vi "GUI_Ch300.vi"() -> ()   [LabVIEW 2013]
uses:
  Shared/GUI_Template/GUI_master/tcp_new_data_event.ctl
  Shared/GUI_Template/GUI_master/tcp new data cluster.ctl
  <vilib>/vision/NI_Vision_Development_Module.lvlib
panel:
  out "tcp data event":T1
  in  "Refresh Button":bool
  in  "localsavingpath::1":path caption="LocalSavingPath"
  in  "STOP":bool
  out "Lineout":dbl[](graph)
  in  "exposure::1":dbl=40.0 caption="Exposure" min=0.0 max=200.0
  in  "ADCGain::1":dbl=1.0 caption="ADC Gain" min=0.0 max=2000.0
  in  "save::1":bool caption="Save"
  in  "trigger::1":T2(ring)=enum."Trigger First (PM only)" caption="Trigger"
  out "image::1":T3(plugin-control) caption="Casca512"
  out "Histogram":T4(graph)
  in  "GUIdevice 1":string="10TW_E-Beam"
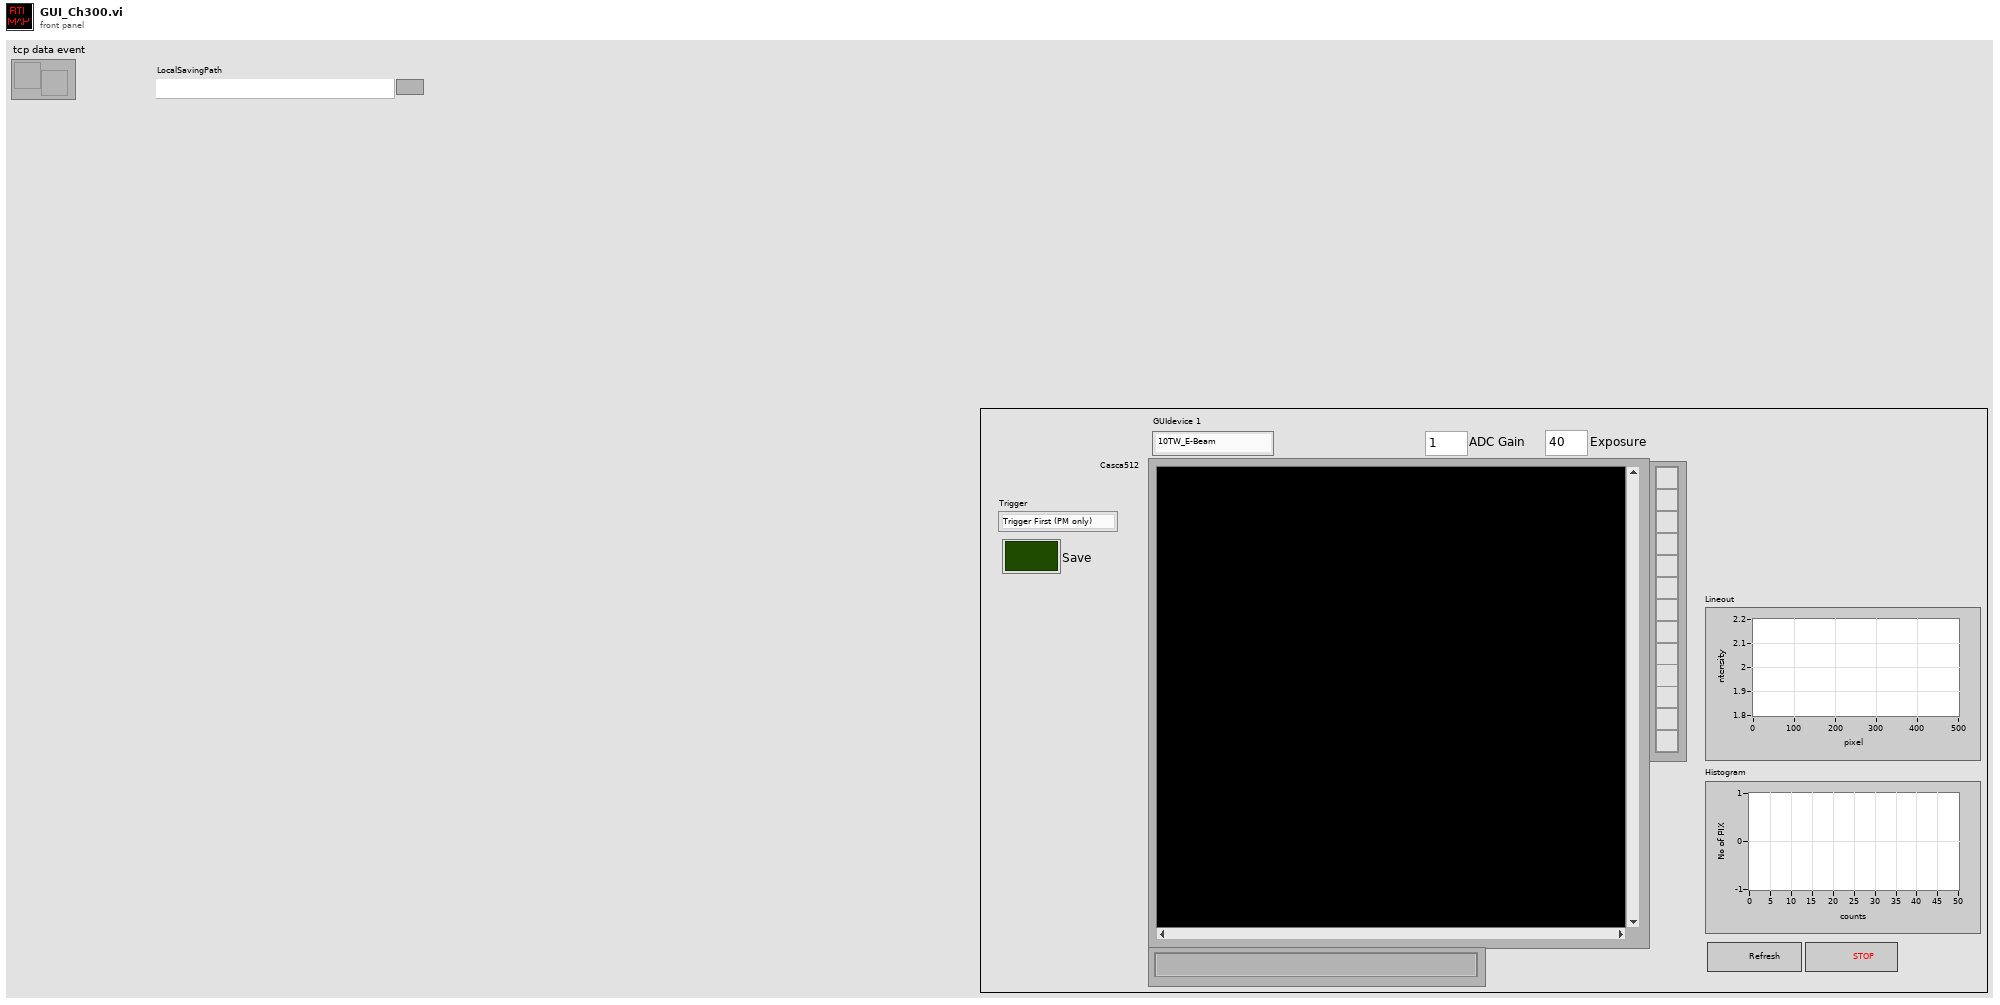
[diagram p1: front panel]
types:
  T1 = typedef "tcp_new_data_event.ctl" = refnum<user-event>
  T2 = enum32{"N/A", "Free Run/Timed", "Trigger First (PM only)", "Ext Sync/Strobed", "Bulb (PM only)", "Variable Exp (PM only)", "Flash Mode (PM only)"}
  T3 = typedef "IMAQ Image.ctl" = refnum<image>
  T4 = cluster{"Starting Value":sgl, "Incremental Value":sgl, "Histogram":u32[]}
  T5 = enum32{"invalid app kind", "Development System", "Run Time System", "Student Edition", "Embedded LabVIEW", "Evaluation", "Custom"}
  T6 = typedef "tcp new data cluster.ctl" = cluster{"EventEnum":enum16{"new data", "connection status update"}, "Device name":string}
  T7 = enum32{"Invalid", "Standard", "Closed", "Hidden", "Minimized", "Maximized"}
  T8 = typedef "Image Type" = u32
  T9 = cluster{"Global Rectangle":i32[], "Contours":cluster{"Contour Type":u32, "ROI Type":u32, "Points":i32[]}[]}
  T10 = typedef "IMAQ Line" = cluster{"Start X":i32, "Start Y":i32, "End X":i32, "End Y":i32}
  T11 = cluster{"Core":cluster{"Current VI Reference":refnum<vi>, "Close Panel on Exit?":bool}, "Your Boolean data":bool, "Your string data":string, "SuperGUI":cluster{"STOP queue":refnum<queue>, "SuperGUI ref":refnum<vi>}}
  T12 = cluster{"STOP queue":refnum<queue>, "SuperGUI ref":refnum<vi>}
  T13 = cluster{"Current VI Reference":refnum<vi>, "Close Panel on Exit?":bool}
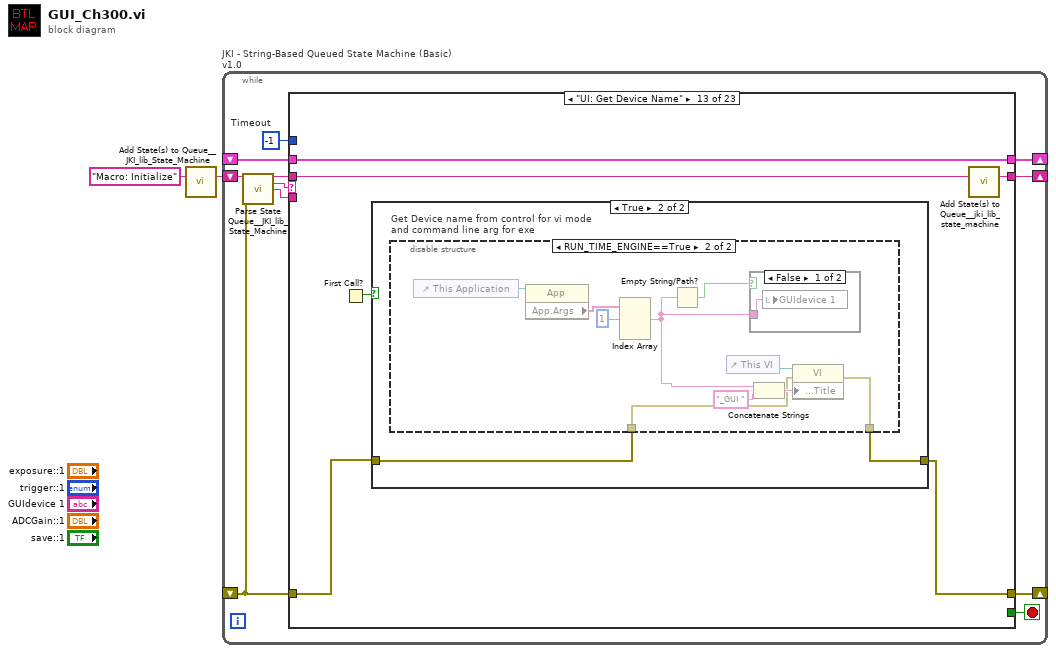
[diagram p0: block diagram]
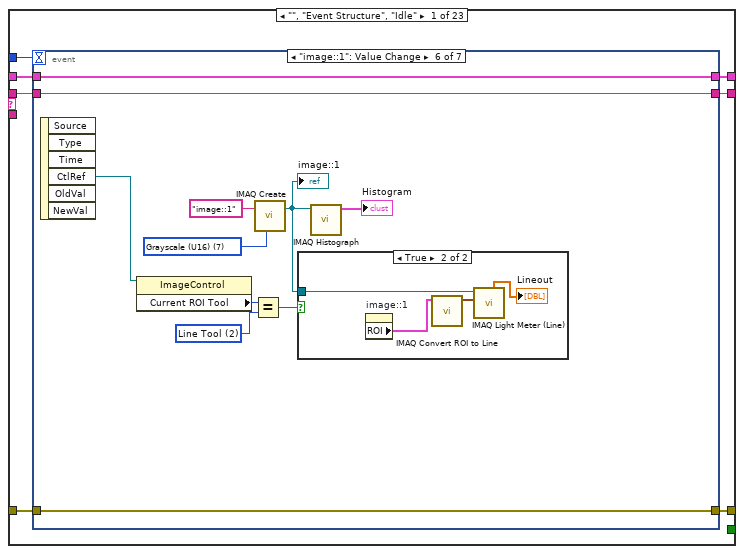
[diagram p2: hidden frame]
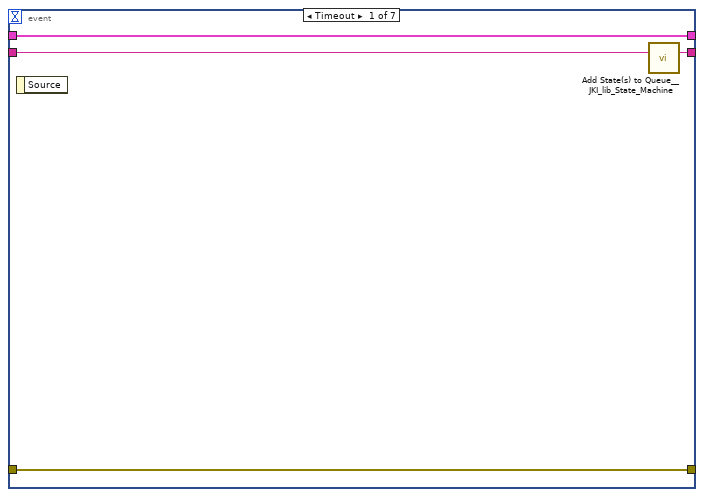
[diagram p3: hidden frame]
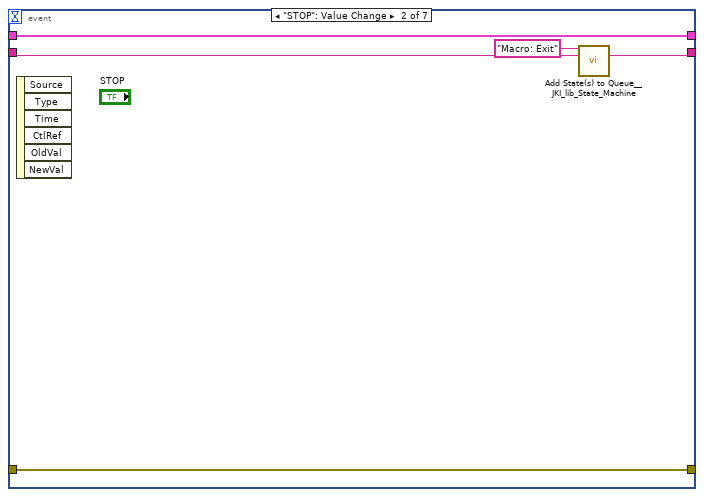
[diagram p4: hidden frame]
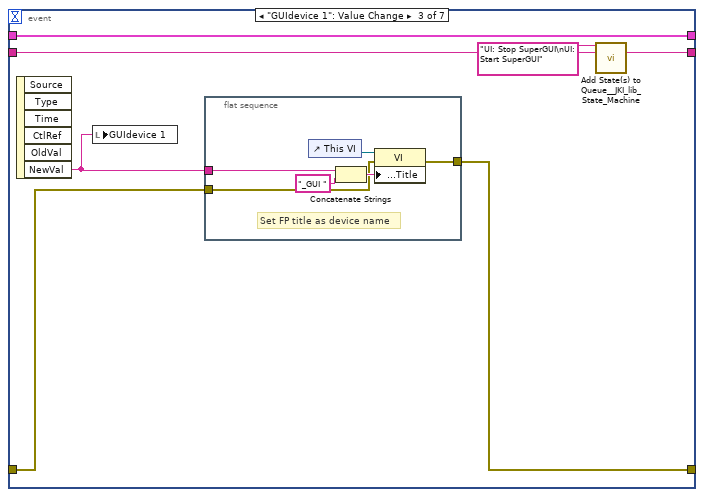
[diagram p5: hidden frame]
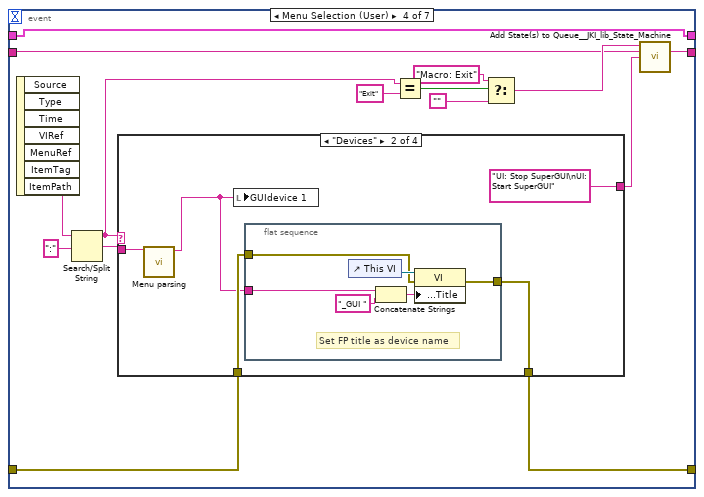
[diagram p6: hidden frame]
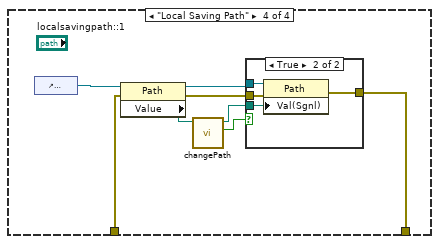
[diagram p9: hidden frame]
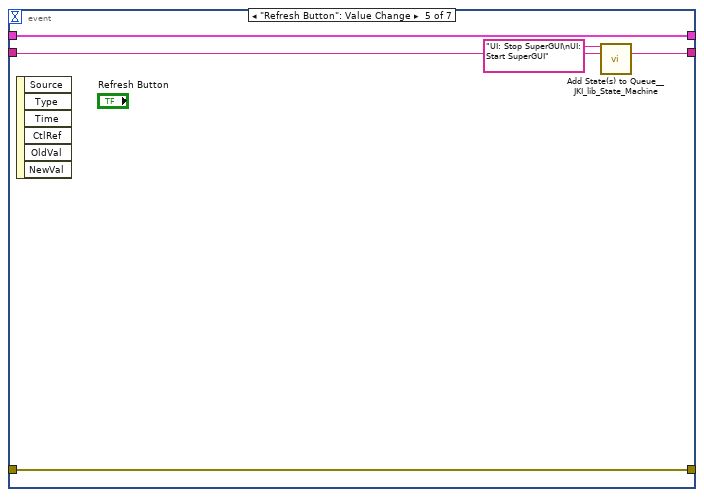
[diagram p11: hidden frame]
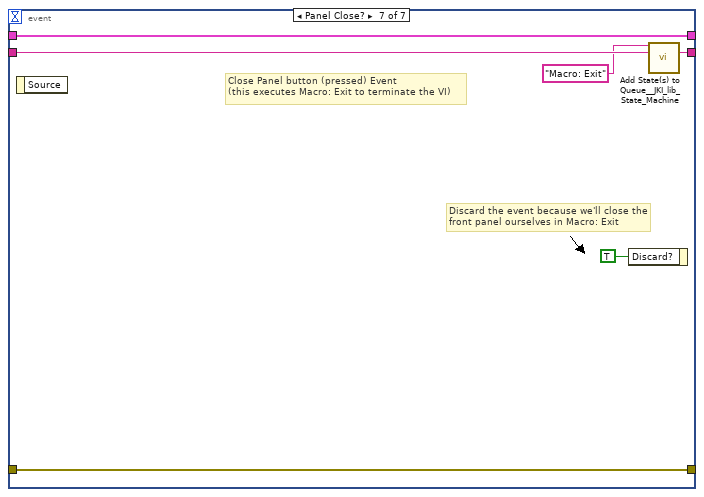
[diagram p13: hidden frame]
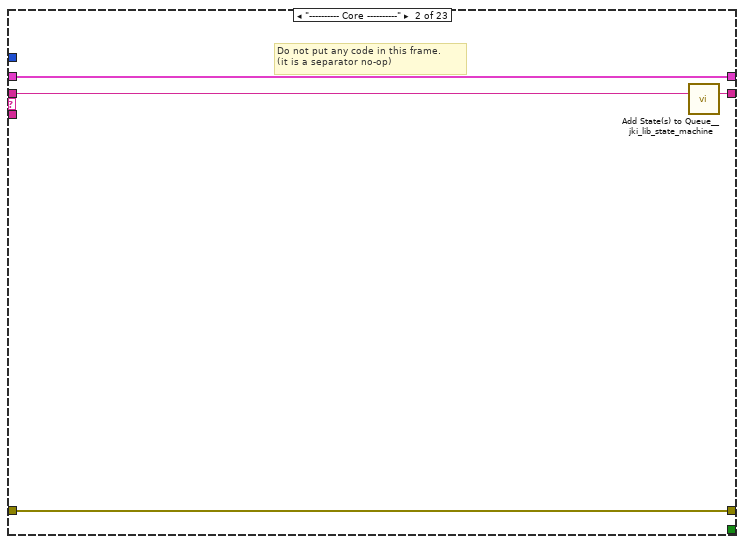
[diagram p14: hidden frame]
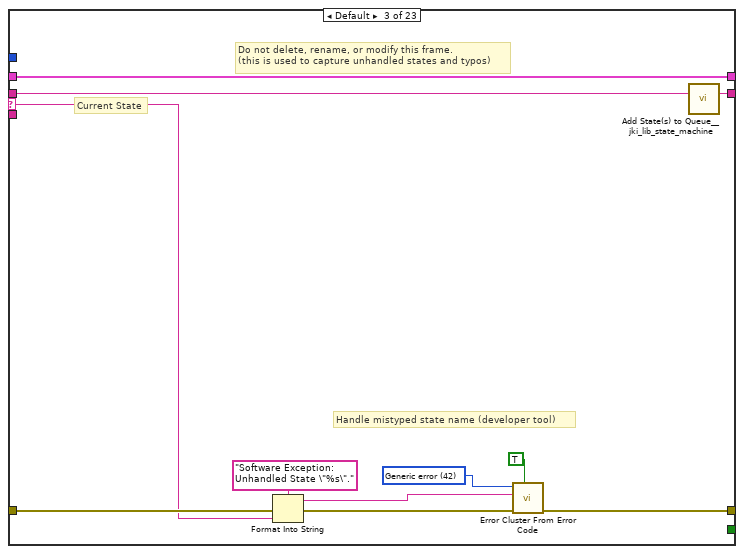
[diagram p15: hidden frame]
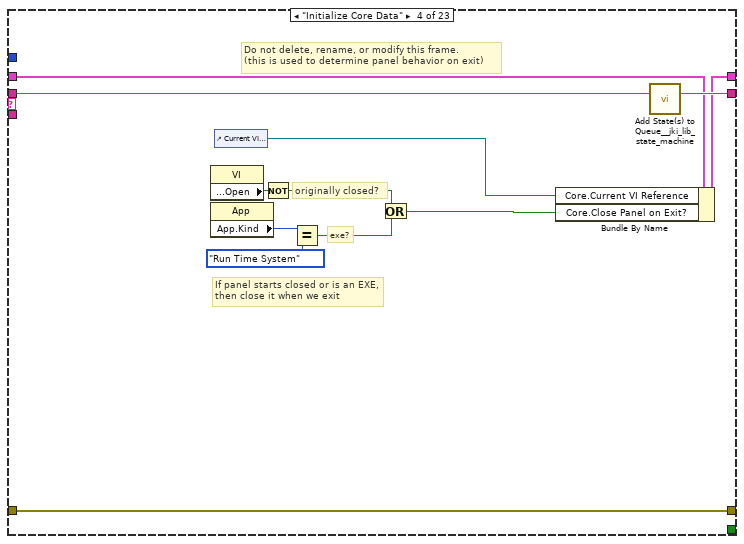
[diagram p16: hidden frame]
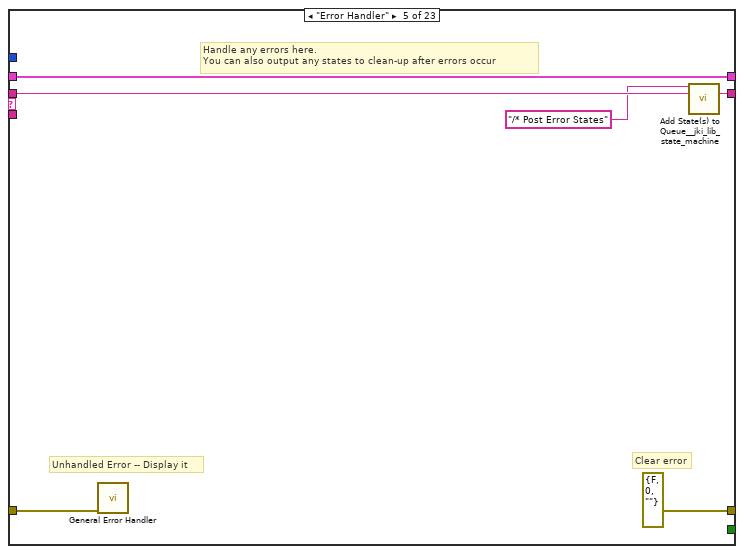
[diagram p17: hidden frame]
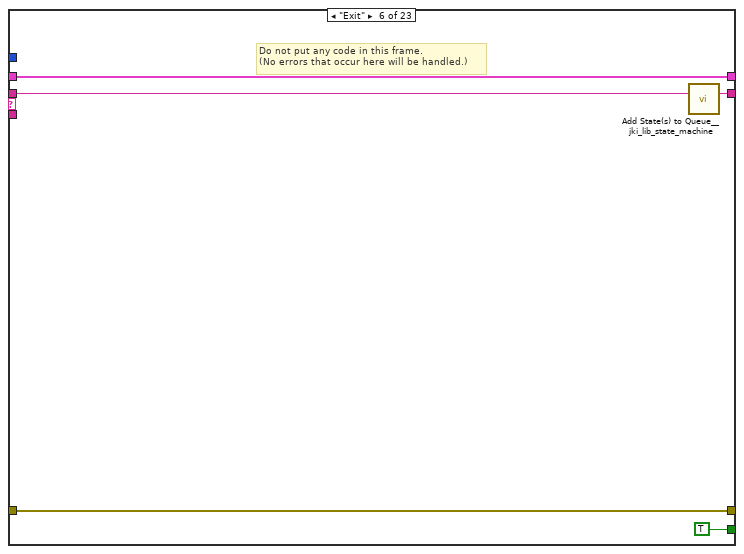
[diagram p18: hidden frame]
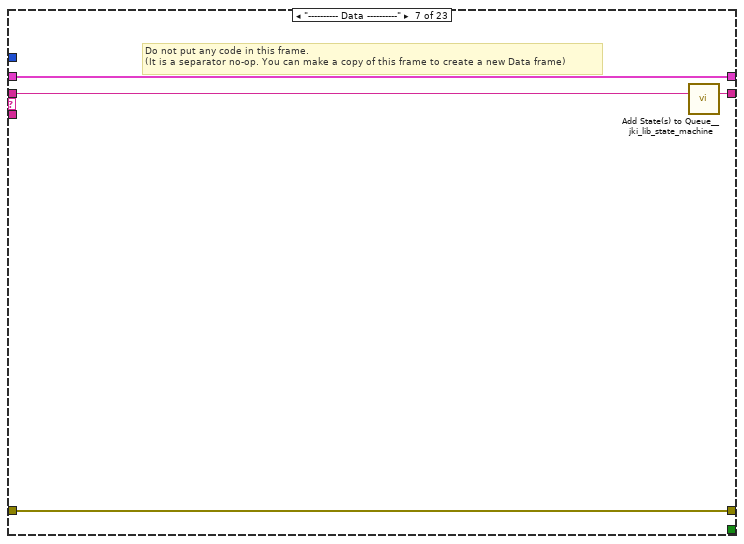
[diagram p19: hidden frame]
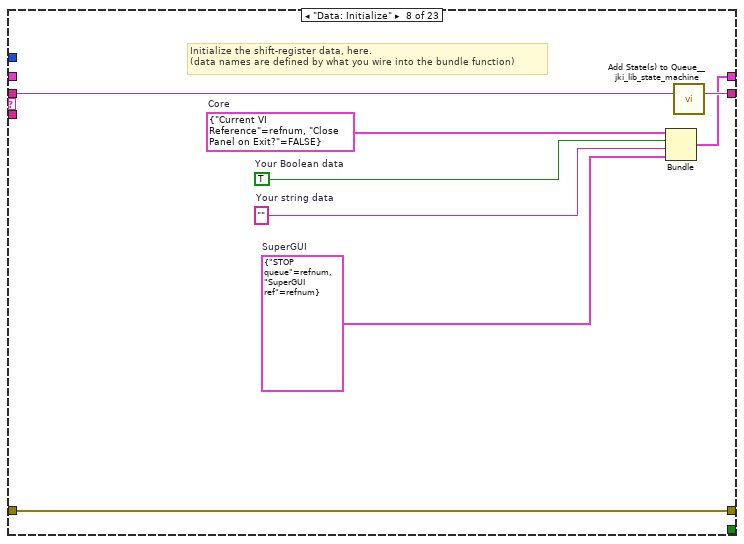
[diagram p20: hidden frame]
diagram:
  n1 = call <vilib>:"Add State(s) to Queue__JKI_lib_State_Machine.vi"("State(s) in (\"\")"="Macro: Initialize") -> ("States Out"=w2:string)  [unwired: 14 in]
  n2 = while "JKI - String-Based Queued State Machine (Basic) v1.0" {
    shift-right: [w6] -> _
    shift-left: _ -> [w5]
    shift-right: [w9] -> _
    shift-left: _ -> [w3]
    shift-right: [w8] -> _
    shift-left: w2 -> [w10]
    stop <- w7 stop-if-true
    w4 = -1  # Timeout
    n3 = call <vilib>:"Parse State Queue__JKI_lib_State_Machine.vi"("State Queue"=w10, "Error In (no error)"=w3) -> ("Remaining States"=w12:string, "Current State"=w13:string, "Arguments"=w11:string)  [unwired: 11 in]
    n4 = case shown="\"UI: Get Device Name\"" w13 {
      selector: w13 -> [_ _ w114 _ _ _ _ _ _ _ _ _ _ _ _ _ _ _ _ _ _ _ _]
      tunnel: w12 -> [w20 w113 w118 w136 w142 w147 w151 w159 w165 w169 w174 w179 w217 w251 w259 w265 w276 w302 w307 w317 w321 w325 w329]
      tunnel: w11 -> [_ _ _ _ _ _ _ _ _ _ _ _ _ _ _ w260 w270 _ _ _ _ _ _]
      tunnel: w5 -> [w18 w110 w116 w127 w139 w145 w148 _ w160 w166 w172 w177 w215 w242 w254 w263 w272 w299 w304 w314 w318 w322 w326]
      tunnel: [w17 w111 w120 w133 errorcluster {"status"=FALSE, "code"=0, "source"=""} ("error out") w144 w149 w156 w161 w167 w170 w175 w212 w235 w252 w261 w273 w300 w305 w315 w319 w323 w327] -> w9
      tunnel: w3 -> [w16 w111 w119 w133 w138 w144 w149 w156 w162 w167 w171 w176 w213 w236 w253 w262 w274 w300 w305 w315 w319 w323 w327]
      tunnel: [w19 w112 w117 w135 w141 w146 w150 w158 w164 w168 w173 w178 w216 w250 w258 w264 w275 w301 w306 w316 w320 w324 w328] -> w8
      tunnel: [_ _ _ _ _ TRUE _ _ _ _ _ _ _ _ _ _ _ _ _ _ _ _ _] -> w7
      tunnel: [w15 w110 w116 w134 w139 w145 w148 w157 w160 w166 w172 w177 w215 w241 w254 w263 w272 w299 w304 w314 w318 w322 w326] -> w6
      tunnel: w4 -> [w14 _ _ _ _ _ _ _ _ _ _ _ _ _ _ _ _ _ _ _ _ _ _]
      frame "", "Event Structure", "Idle" {
        n5 = event shown="[5] \"image::1\": Value Change" {
          selector: _ -> [_ _ _ _ _ _ _]
          dyn-events: _ -> [_ _ _ _ _ _ _]
          timeout: w14 -> [_ _ _ _ _ _ _]
          tunnel: w20 -> [w24 w27 w33 w51 w86 w98 w109]
          tunnel: [w23 w26 w32 w50 w85 w98 w108] -> w19
          tunnel: w18 -> [w21 w29 w36 w57 w88 w99 w106]
          tunnel: [w22 w28 w34 w44 w87 w97 w107] -> w17
          tunnel: w16 -> [w22 w28 w35 w45 w87 w97 w107]
          tunnel: [w21 w29 w36 w57 w88 w99 w106] -> w15
          event Timeout {
            n6 = event-data() -> ()  [unwired: 1 in, 1 out]
            n7 = call <vilib>:"Add State(s) to Queue__JKI_lib_State_Machine.vi"("State(s) in (\"\")"=w24) -> ("States Out"=w23:string)  [unwired: 14 in]
          }
          event "STOP": Value Change {
            n8 = event-data() -> ()  [unwired: 1 in, 6 out]
            n9 = call <vilib>:"Add State(s) to Queue__JKI_lib_State_Machine.vi"("State(s) in Front (\"\")"="Macro: Exit", "State(s) in (\"\")"=w27) -> ("States Out"=w26:string)  [unwired: 13 in]
          }
          event "GUIdevice 1": Value Change {
            n10 = event-data() -> ("NewVal"=w30:string)  [unwired: 1 in, 5 out]
            n11 = local write "GUIdevice 1"(w30) -> ()
            n12 = flat-sequence {
              tunnel: [w39] -> w34
              tunnel: w35 -> [w38]
              tunnel: w30 -> [w37]
              frame #0 {
                # "Set FP title as device name"
                n13 = control-ref of="This VI"() -> (w42:refnum<vi>)
                n14 = Concatenate Strings(w37, "_GUI ") -> (w41:string)
                n15 = property class="VI"(reference=w42, error in=w38, "Front Panel.Title"=w41) -> (error out=w39:errorcluster)  [unwired: 1 out]
              }
            }
            n16 = call <vilib>:"Add State(s) to Queue__JKI_lib_State_Machine.vi"("State(s) in Front (\"\")"="UI: Stop SuperGUI\nUI: Start SuperGUI", "State(s) in (\"\")"=w33) -> ("States Out"=w32:string)  [unwired: 13 in]
          }
          event Menu Selection (User) {
            n17 = event-data() -> ("ItemPath"=w47:string)  [unwired: 1 in, 6 out]
            n18 = Search/Split String(string=w47, search string/char (-)=":") -> (substring before match=w43:string, match + rest of string=w46:string)  [unwired: 1 in, 1 out]
            n19 = case shown="\"Devices\"" w43 {
              tunnel: w46 -> [_ w63 _ _]
              tunnel: w45 -> [w58 w62 w70 w73]
              tunnel: [w58 w61 w70 w72] -> w44
              tunnel: [_ "UI: Stop SuperGUI\nUI: Start SuperGUI" _ _] -> w49
              frame "", Default {
              }
              frame "Devices" {
                n20 = call "Menu parsing.vi"("ItemPath"=w63) -> ("ItemPath"=w59:string)  [unwired: 9 in, 1 out]
                n21 = local write "GUIdevice 1"(w59) -> ()
                n22 = flat-sequence {
                  tunnel: [w66] -> w61
                  tunnel: w62 -> [w65]
                  tunnel: w59 -> [w64]
                  frame #0 {
                    # "Set FP title as device name"
                    n23 = control-ref of="This VI"() -> (w69:refnum<vi>)
                    n24 = Concatenate Strings(w64, "_GUI ") -> (w68:string)
                    n25 = property class="VI"(reference=w69, error in=w65, "Front Panel.Title"=w68) -> (error out=w66:errorcluster)  [unwired: 1 out]
                  }
                }
              }
              frame "Exit" {
              }
              frame "Local Saving Path" {
                n26 = control-ref of="localsavingpath::1"() -> (w74:refnum<vi>)
                n27 = property class="Path"(reference=w74, error in=w73) -> (reference out=w76:refnum<vi>, error out=w71:errorcluster, "Value"=w75:path)
                n28 = call "changePath.vi"("Local Saving in (h)"=w75) -> ("change (h)"=w77:bool, "Local Saving out (h)"=w78:path)  [unwired: 9 in]
                n29 = case shown="True" w77 {
                  tunnel: w76 -> [_ w83]
                  tunnel: w78 -> [_ w82]
                  tunnel: [w79 w81] -> w72
                  tunnel: w71 -> [w79 w80]
                  frame False {
                  }
                  frame True {
                    n30 = property class="Path"(reference=w83, error in=w80, "Val(Sgnl)"=w82) -> (error out=w81:errorcluster)  [unwired: 1 out]
                  }
                }
              }
            }
            n31 = Equal?(x=w43, y="Exit") -> (x = y?=w55:bool)
            n32 = Select(t="Macro: Exit", s=w55, f="") -> (s? t:f=w52:string)
            n33 = call <vilib>:"Add State(s) to Queue__JKI_lib_State_Machine.vi"("State(s) in Front (\"\")"=w52, "State(s) in (\"\")"=w51, "State(s) at Back (\"\")"=w49) -> ("States Out"=w50:string)  [unwired: 12 in]
          }
          event "Refresh Button": Value Change {
            n34 = event-data() -> ()  [unwired: 1 in, 6 out]
            n35 = call <vilib>:"Add State(s) to Queue__JKI_lib_State_Machine.vi"("State(s) in Front (\"\")"="UI: Stop SuperGUI\nUI: Start SuperGUI", "State(s) in (\"\")"=w86) -> ("States Out"=w85:string)  [unwired: 13 in]
          }
          event "image::1": Value Change {
            w94 = u32 2 items=["Zoom Tool"=8, "Selection Tool"=0, "Pan Tool"=9, "Point Tool"=1, "Line Tool"=2, "Rectangle Tool"=3, "Rotated Rectangle Tool"=12, "Polyline Tool"=10, "Polygon Tool"=5, "Freehand Tool"=11, "Closed Freehand Tool"=6, "Ellipse Tool"=4, "Annulus Tool"=7] ("Current ROI Tool")
            w91 = T8 7 items=["Grayscale (U8)", "Grayscale (I16)", "Grayscale (SGL)", "Complex (CSG)", "RGB (U32)", "HSL (U32)", "RGB (U64)", "Grayscale (U16)"] ("Image Type")
            n36 = event-data() -> ("CtlRef"=w89:refnum<vi>)  [unwired: 1 in, 5 out]
            n37 = property on="Property Node" class="ImageControl"(reference=w89) -> ("Current ROI Tool"=w93:u32)  [unwired: 1 in, 2 out]
            n38 = Equal?(x=w93, y=w94) -> (x = y?=w95:bool)
            n39 = call "IMAQ Create"("Image Name"="image::1", "Image Type"=w91) -> ("New Image"=w96:T3)  [unwired: 3 in, 1 out]
            "image::1" <- w96
            n40 = case shown="True" w95 {
              tunnel: w96 -> [_ w101]
              frame False {
              }
              frame True {
                n41 = property on="image::1" class="ImageControl"() -> ("ROI"=w103:T9)  [unwired: 2 in, 2 out]
                n42 = call "IMAQ Convert ROI to Line"("ROI Descriptor"=w103) -> ("Line"=w102:T10)  [unwired: 8 in, 1 out]
                n43 = call "IMAQ Light Meter (Line)"("Line"=w102, "Image"=w101) -> ("Line Profile"=→"Lineout":dbl[])  [unwired: 5 in, 4 out]
              }
            }
            n44 = call "IMAQ Histograph"("Image"=w96) -> ("Histogram Graph"=→"Histogram":T4)  [unwired: 7 in, 3 out]
          }
          event Panel Close? {
            # "Discard the event because we'll close the front panel ourselves in Macro: Exit"
            # "Close Panel button (pressed) Event\n(this executes Macro: Exit to terminate the VI)"
            n45 = event-data() -> ()  [unwired: 1 in, 1 out]
            n46 = event-data("Discard?"=TRUE) -> ()  [unwired: 1 in, 1 out]
            n47 = call <vilib>:"Add State(s) to Queue__JKI_lib_State_Machine.vi"("State(s) in Front (\"\")"="Macro: Exit", "State(s) in (\"\")"=w109) -> ("States Out"=w108:string)  [unwired: 13 in]
          }
        }
      }
      frame "---------- Core ----------" {
        # "Do not put any code in this frame.\n(it is a separator no-op)"
        n48 = call <vilib>:"Add State(s) to Queue__jki_lib_state_machine.vi"("State(s) in (\"\")"=w113) -> ("States Out"=w112:string)  [unwired: 14 in]
      }
      frame Default {
        w123 = 42 items=["No error", "Argument error", "Memory is full", "Out of zone", "End of file", "File already open", "Generic file I/O error", "File not found", "File permission error", "Disk is full", "Duplicate path", "Too many files open", "System feature not enabled", "Resource file not found", "Cannot add resource", "Resource not found", "Image not found", "Image memory error", "Pen does not exist", "Config type invalid", "Config token not found", "Config parse error", "Config memory error", "Bad external code format", "Bad external code offset", "External code not present", "Null window", "Destroy window error", "Null menu", "Print aborted", "Bad print record", "Print driver error", "Windows error during printing", "Memory error during printing", "Print dialog error", "Generic print error", "Invalid device refnum", "Device not found", "Device parameter error", "Device unit error", "Cannot open device", "Device call aborted", "Generic error", "Cancelled by user", "Object ID too low", "Object ID too high", "Object not in heap", "Unknown heap", "Unknown object (invalid DefProc)", "Unknown object (DefProc not in table)", "Message out of range", "Invalid (null) method", "Unknown message", "Manager call not supported", "Bad address", "Network operation in progress", "Network operation timed out", "Connection is busy", "Network attribute not supported", "Network error", "Address in use", "System out of memory", "Connection aborted", "Connection refused", "Not connected", "Already connected", "Connection closed", "Initialization error (interapplication manager)", "Bad occurrence", "Wait on unbound occurrence handler", "Occurrence queue overflow", "Datalog type conflict", "Unused", "Unrecognized type (interapplication manager)", "Memory corrupt", "Failed to make temporary DLL", "Old CIN version", "Drag socket not found", "Failed to load drop-object", "Failed to register OLE object", "Failed to release OLE object", "Format specifier type mismatch", "Unknown format specifier", "Too few format specifiers", "Too many format specifiers", "Scan failed", "Newer CIN version", "Error converting to variant", "Runtime menu error", "Password tampered", "Variant attribute not found", "Incompatible variant data type", "Event data is not available", "Event Store is not present", "Occurrence is not found", "Event Queue is not created", "Event info is not available", "Refnum passed is NULL", "Error retrieving Class GUID", "Error retrieving CoClass GUID", "Error retrieving TypeLib GUID.", "Bad built application magic bytes.", "Specific driver is different from the specific driver associated with the Logical Name.", "There is no session opened to the class driver.", "Max Error", "MAX - Error with config objects", "MAX - Error loading configuration", "MAX - Group not supported"]
        # "Current State"
        # "Do not delete, rename, or modify this frame.\n(this is used to capture unhandled states and typos)"
        # "Handle mistyped state name (developer tool)"
        n49 = Format Into String(format string="Software Exception: Unhandled State \"%s\"." ("message"), error in=w119, w114) -> (resulting string=w122:string, error out=w121:errorcluster)  [unwired: 1 in]
        n50 = call <vilib>:"Error Cluster From Error Code.vi"("show call chain? (False)"=TRUE, "error in (no error)"=w121, "error message (\"\")"=w122, "error code (0)"=w123) -> ("error out"=w120:errorcluster)  [unwired: 5 in]
        n51 = call <vilib>:"Add State(s) to Queue__jki_lib_state_machine.vi"("State(s) in (\"\")"=w118) -> ("States Out"=w117:string)  [unwired: 14 in]
      }
      frame "Initialize Core Data" {
        # "Do not delete, rename, or modify this frame.\n(this is used to determine panel behavior on exit)"
        # "originally closed?"
        # "exe?"
        # "If panel starts closed or is an EXE, then close it when we exit"
        n52 = property class="VI"() -> ("Front Panel.Open"=w132:bool)  [unwired: 2 in, 2 out]
        n53 = property class="App"() -> ("App.Kind"=w131:T5)  [unwired: 2 in, 2 out]
        n54 = control-ref of="Current VI Reference"() -> (w125:refnum<vi>)
        n55 = Not(x=w132) -> (.not. x?=w129:bool)
        n56 = Equal?(x=w131, y=T5."Run Time System" ("Application:Kind")) -> (x = y?=w128:bool)
        n57 = Or(x=w129, y=w128) -> (x .or. y?=w126:bool)
        n58 = Bundle By Name(cluster=w127, "Core.Current VI Reference"=w125, "Core.Close Panel on Exit?"=w126) -> (w134:T11)
        n59 = call <vilib>:"Add State(s) to Queue__jki_lib_state_machine.vi"("State(s) in (\"\")"=w136) -> ("States Out"=w135:string)  [unwired: 14 in]
      }
      frame "Error Handler" {
        # "Unhandled Error -- Display it"
        # "Handle any errors here.\nYou can also output any states to clean-up after errors occur"
        # "Clear error"
        n60 = call <vilib>:"General Error Handler.vi"("error in (no error)"=w138) -> ()  [unwired: 10 in, 5 out]
        n61 = call <vilib>:"Add State(s) to Queue__jki_lib_state_machine.vi"("State(s) in Front (\"\")"="/* Post Error States", "State(s) in (\"\")"=w142) -> ("States Out"=w141:string)  [unwired: 13 in]
      }
      frame "Exit" {
        # "Do not put any code in this frame.\n(No errors that occur here will be handled.)"
        n62 = call <vilib>:"Add State(s) to Queue__jki_lib_state_machine.vi"("State(s) in (\"\")"=w147) -> ("States Out"=w146:string)  [unwired: 14 in]
      }
      frame "---------- Data ----------" {
        # "Do not put any code in this frame.\n(It is a separator no-op. You can make a copy of this frame to create a new Data frame)"
        n63 = call <vilib>:"Add State(s) to Queue__jki_lib_state_machine.vi"("State(s) in (\"\")"=w151) -> ("States Out"=w150:string)  [unwired: 14 in]
      }
      frame "Data: Initialize" {
        w152 = T12 {"STOP queue"=refnum, "SuperGUI ref"=refnum}  # SuperGUI
        w153 = T13 {"Current VI Reference"=refnum, "Close Panel on Exit?"=FALSE}  # Core
        w155 = TRUE  # Your Boolean data
        w154 = ""  # Your string data
        # "Initialize the shift-register data, here.\n(data names are defined by what you wire into the bundle function)"
        n64 = Bundle("Core"=w153, "Your Boolean data"=w155, "Your string data"=w154, "SuperGUI"=w152) -> (w157:T11)  [unwired: 1 in]
        n65 = call <vilib>:"Add State(s) to Queue__jki_lib_state_machine.vi"("State(s) in (\"\")"=w159) -> ("States Out"=w158:string)  [unwired: 14 in]
      }
      frame "Data: Cleanup" {
        # "Cleanup any data and references, here.\n(this is called automatically, by the Macro: Exit)"
        n66 = Unbundle By Name(w160) -> ("Core.Current VI Reference"=w163:refnum<vi>)
        n67 = Close Reference(reference=w163, error in (no error)=w162) -> (error out=w161:errorcluster)
        n68 = call <vilib>:"Add State(s) to Queue__jki_lib_state_machine.vi"("State(s) in (\"\")"=w165) -> ("States Out"=w164:string)  [unwired: 14 in]
      }
      frame "---------- UI ----------" {
        # "Do not put any code in this frame.\n(It is a separator no-op. You can make a copy of this frame to create a new UI frame)"
        n69 = call <vilib>:"Add State(s) to Queue__jki_lib_state_machine.vi"("State(s) in (\"\")"=w169) -> ("States Out"=w168:string)  [unwired: 14 in]
      }
      frame "UI: Initialize" {
        # "Initialize the User Interface, here.\n(this is called automatically, by the Macro: Init)"
        n70 = call <userlib>:"Fit VI window to Largest Dec__ogtk.vi"("error in (no error)"=w171) -> ("error out"=w170:errorcluster)  [unwired: 5 in, 1 out]
        n71 = call <vilib>:"Add State(s) to Queue__jki_lib_state_machine.vi"("State(s) in (\"\")"=w174) -> ("States Out"=w173:string)  [unwired: 14 in]
      }
      frame "UI: Update Device List" {
        n72 = disable-structure shown="Disabled" {
          disable-tunnel: w176 -> [w184 w211]
          disable-tunnel: [w182 w211] -> w175
          frame Disabled {
            n73 = call "getDevices.vi"("Device Class"="") -> ("All Devices"=w180:string[])
            n74 = Empty Array?(array=w180) -> (empty?=w181:bool)
            n75 = case shown="False" w181 {
              tunnel: w184 -> [w187 w210]
              tunnel: [w186 w210] -> w182
              tunnel: w180 -> [w185 _]
              frame False {
                n76 = Current VI's Menubar() -> (w190:refnum<k9>)
                n77 = Get Menu Item Info(7:"Devices" ("item tag"), 8:w187, 11:w190) -> (0:w196:errorcluster, 3:w192:refnum<k9>)  [unwired: 5 out]
                n78 = Set Menu Item Info(7:"Devices" ("item tag"), 8:w196, 9:TRUE ("enabled"), 11:w192) -> (0:w195:errorcluster, 3:w194:refnum<k9>)  [unwired: 3 in]
                n79 = First Call?() -> (First Call?: T/F=w188:bool)
                n80 = case shown="True" w188 {
                  tunnel: w194 -> [_ w202]
                  tunnel: w185 -> [_ w201]
                  tunnel: w195 -> [w197 w199]
                  tunnel: [w197 w198] -> w186
                  frame False {
                  }
                  frame True {
                    n81 = for {
                      tunnel: [w209] -> w203
                      tunnel: w201 -> [w207] mode=indexing
                      tunnel: w202 -> [w206]
                      tunnel: [w205] -> w200
                      tunnel: w199 -> [w204]
                      n82 = Insert Menu Items(5:"Devices" ("menu tag"), 6:w204, 7:w207, 8:w207, 9:w206) -> (0:w205:errorcluster, 3:w209:refnum<k9>)  [unwired: 1 in, 1 out]
                    }
                    n83 = Enable Menu Tracking(2:w200, 4:w203) -> (0:w198:errorcluster)  [unwired: 1 in, 1 out]
                  }
                }
              }
              frame True {
              }
            }
          }
          frame Enabled {
          }
        }
        n84 = call <vilib>:"Add State(s) to Queue__jki_lib_state_machine.vi"("State(s) in (\"\")"=w179) -> ("States Out"=w178:string)  [unwired: 14 in]
      }
      frame "UI: Get Device Name" {
        n85 = First Call?() -> (First Call?: T/F=w214:bool)
        n86 = case shown="True" w214 {
          tunnel: w213 -> [w218 w220]
          tunnel: [w218 w219] -> w212
          frame False {
          }
          frame True {
            n87 = disable-structure "Get Device name from control for vi mode\nand command line arg for exe" shown="RUN_TIME_ENGINE==True" {
              disable-tunnel: w220 -> [_ w222]
              disable-tunnel: [_ w221] -> w219
              frame condition #0 (active) {
              }
              frame condition #1 {
                n88 = control-ref of="This Application"() -> (w230:refnum<vi>)
                n89 = property class="App"(reference=w230) -> ("App.Args"=w229:string[])  [unwired: 1 in, 2 out]
                n90 = Index Array(array=w229, index #1=1 ("index")) -> (element #1=w223:string)  [unwired: 2 in, 2 out]
                n91 = Empty String/Path?(string/path=w223) -> (empty?=w227:bool)
                n92 = control-ref of="This VI"() -> (w226:refnum<vi>)
                n93 = case shown="False" w227 {
                  tunnel: w223 -> [w231 _]
                  frame False {
                    n94 = local write "GUIdevice 1"(w231) -> ()
                  }
                  frame True {
                  }
                }
                n95 = Concatenate Strings(w223, "_GUI ") -> (w225:string)
                n96 = property class="VI"(reference=w226, error in=w222, "Front Panel.Title"=w225) -> (error out=w221:errorcluster)  [unwired: 1 out]
              }
            }
          }
        }
        n97 = call <vilib>:"Add State(s) to Queue__jki_lib_state_machine.vi"("State(s) in (\"\")"=w217) -> ("States Out"=w216:string)  [unwired: 14 in]
      }
      frame "UI: Start SuperGUI" {
        # "create stop queue for supergui and its clones"
        # "x100 abort will be dependent on caller VI\nx80 abort will be independent of caller vi, this will abort vi when labview is closed."
        # "Start SuperGUI asynchronous way"
        n98 = vi-ref "GUI_Master_subvi_reentrant_queues.vi"() -> (w234:refnum<vi>)
        n99 = property class="VI"(reference=w234) -> ("Path"=w233:path)  [unwired: 1 in, 2 out]
        n100 = Create User Event(user event datatype=T6 {"EventEnum"=enum."new data", "Device name"="Device name"} ("New Event"), error in=w236) -> (user event=w237:refnum<user-event>, error out=w243:errorcluster)
        "tcp data event" <- w237
        n101 = control-ref of="This Application"() -> (w240:refnum<vi>)
        n102 = control-ref of="This VI"() -> (w239:refnum<vi>)
        n103 = Open VI Reference(type specifier VI Refnum (for type only)=refnum<vi> refnum, vi path=w233, options=256) -> (vi reference=w249:refnum<vi>, error out=w248:errorcluster)  [unwired: 3 in]
        n104 = register-events(w237) -> ()  [unwired: 2 in, 2 out]
        n105 = call "supergui create stop queue.vi"() -> ("STOP Queue out"=w245:refnum<queue>)  [unwired: 11 in]
        n106 = Current VI's Menubar() -> (w238:refnum<k9>)
        n107 = call-by-ref "Start Asynchronous Call"(reference=w249, error in=w248, "STOP Queue in"=w245, "This Application"=w240, 8:"error in (no error)"=w243, "tcp data event"=w237, "Caller menu reference"=w238, "Caller VI ref"=w239) -> (reference out=w232:refnum<vi>, error out=w235:errorcluster)  [unwired: 5 in, 1 out]
        n108 = Bundle By Name(cluster=w242, "SuperGUI.SuperGUI ref"=w232, "SuperGUI.STOP queue"=w245) -> (w241:T11)
        n109 = call <vilib>:"Add State(s) to Queue__jki_lib_state_machine.vi"("State(s) in (\"\")"=w251) -> ("States Out"=w250:string)  [unwired: 14 in]
      }
      frame "UI: Stop SuperGUI" {
        # "Stop Supergui Clone and wait until it exit properly"
        n110 = Unbundle By Name(w254) -> ("SuperGUI.SuperGUI ref"=w256:refnum<vi>, "SuperGUI.STOP queue"=w255:refnum<queue>)
        n111 = Release Queue(queue=w255, error in (no error)=w253) -> (error out=w257:errorcluster)  [unwired: 1 in, 2 out]
        n112 = call-by-ref "Wait On Asynchronous Call"(reference=w256, error in=w257) -> ("error out"=w252:errorcluster)  [unwired: 11 in, 2 out]
        n113 = call <vilib>:"Add State(s) to Queue__jki_lib_state_machine.vi"("State(s) in (\"\")"=w259) -> ("States Out"=w258:string)  [unwired: 14 in]
      }
      frame "UI: Cursor Set" {
        # "Argument"
        # "Set and Unset Cursor Busy.\n(Usage: \"UI: Cursor Set >> Busy|Idle\")"
        n114 = case shown="\"Idle\", Default" w260 {
          tunnel: w262 -> [w267 w269]
          tunnel: [w266 w268] -> w261
          frame "Idle", Default {
            n115 = call <vilib>:"Unset Busy.vi"("error in (no error)"=w267) -> ("error out"=w266:errorcluster)  [unwired: 10 in]
          }
          frame "Busy" {
            n116 = call <vilib>:"Set Busy.vi"("error in (no error)"=w269) -> ("error out"=w268:errorcluster)  [unwired: 9 in, 1 out]
          }
        }
        n117 = call <vilib>:"Add State(s) to Queue__jki_lib_state_machine.vi"("State(s) in (\"\")"=w265) -> ("States Out"=w264:string)  [unwired: 14 in]
      }
      frame "UI: Front Panel State" {
        # "Argument"
        # "Set Front Panel Open or Closed\n(Usage: \"UI: Front Panel State >> Open|Close\")"
        n118 = Unbundle By Name(w272) -> ("Core.Current VI Reference"=w271:refnum<vi>)
        n119 = case shown="\"Open\", Default" w270 {
          tunnel: w274 -> [w280 w293]
          tunnel: [w282 w294] -> w273
          tunnel: w271 -> [w281 w291]
          frame "Open", Default {
            n120 = property class="VI"(reference=w281, error in=w280) -> (reference out=w278:refnum<vi>, error out=w279:errorcluster, "Front Panel.Open"=w277:bool)
            n121 = case shown="False" w277 {
              tunnel: [w285 w288] -> w282
              tunnel: w279 -> [w284 w288]
              tunnel: w278 -> [w283 _]
              frame False {
                n122 = invoke class="VI" method="FP.Open"(reference=w283, error in=w284, "Activate"=TRUE, "State"=T7."Standard") -> (error out=w285:errorcluster)  [unwired: 1 in, 4 out]
              }
              frame True {
              }
            }
          }
          frame "Close" {
            n123 = property class="VI"(reference=w291, error in=w293) -> (reference out=w290:refnum<vi>, error out=w292:errorcluster, "Front Panel.Open"=w289:bool)
            n124 = case shown="True" w289 {
              tunnel: [w295 w298] -> w294
              tunnel: w292 -> [w295 w297]
              tunnel: w290 -> [_ w296]
              frame False {
              }
              frame True {
                n125 = invoke class="VI" method="FP.Close"(reference=w296, error in=w297) -> (error out=w298:errorcluster)  [unwired: 1 in, 2 out]
              }
            }
          }
        }
        n126 = call <vilib>:"Add State(s) to Queue__jki_lib_state_machine.vi"("State(s) in (\"\")"=w276) -> ("States Out"=w275:string)  [unwired: 14 in]
      }
      frame "---------- Macro ----------" {
        # "Do not put any code in this frame.\n(It is a separator no-op. You can make a copy of this frame to create a new Macro frame)"
        n127 = call <vilib>:"Add State(s) to Queue__jki_lib_state_machine.vi"("State(s) in (\"\")"=w302) -> ("States Out"=w301:string)  [unwired: 14 in]
      }
      frame "Macro: Initialize" {
        # "Initialization Macro\n(This is called once, when the VI starts)"
        n128 = call <vilib>:"Add State(s) to Queue__jki_lib_state_machine.vi"("State(s) in Front (\"\")"="Data: Initialize\nInitialize Core Data\nUI: Initialize\nUI: Update Device List\nUI: Get Device Name\nUI: Start SuperGUI\nUI: Front Panel State >> Open", "State(s) in (\"\")"=w307) -> ("States Out"=w306:string)  [unwired: 13 in]
      }
      frame "Macro: Exit" {
        # "Exit Macro\n(This is called once, when the VI exits)"
        n129 = Unbundle By Name(w314) -> ("Core.Close Panel on Exit?"=w313:bool)
        n130 = Select(t="UI: Front Panel State >> Close", s=w313, f="") -> (s? t:f=w310:string)
        n131 = call <vilib>:"Add State(s) to Queue__jki_lib_state_machine.vi"("State(s) in (\"\")"=w310, "State(s) at Back (\"\")"="Data: Cleanup\nExit") -> ("States Out"=w308:string)  [unwired: 13 in]
        n132 = call <vilib>:"Add State(s) to Queue__jki_lib_state_machine.vi"("State(s) in Front (\"\")"=w308, "State(s) in (\"\")"=w317) -> ("States Out"=w316:string)  [unwired: 13 in]
      }
      frame "---------- New Category ----------" {
        # "Template Separator\n(You can make a copy of, or modify, this frame)"
        n133 = call <vilib>:"Add State(s) to Queue__jki_lib_state_machine.vi"("State(s) in (\"\")"=w321) -> ("States Out"=w320:string)  [unwired: 14 in]
      }
      frame "New Category: 1" {
        # "Your code here.\n(You can make a copy of, or modify, this frame)"
        n134 = call <vilib>:"Add State(s) to Queue__jki_lib_state_machine.vi"("State(s) in (\"\")"=w325) -> ("States Out"=w324:string)  [unwired: 14 in]
      }
      frame "New Category: 2" {
        # "Your code here.\n(You can make a copy of, or modify, this frame)"
        n135 = call <vilib>:"Add State(s) to Queue__jki_lib_state_machine.vi"("State(s) in (\"\")"=w329) -> ("States Out"=w328:string)  [unwired: 14 in]
      }
    }
  }
